vi "ThermoV_ControlSweep_2VO_160718.vi"() -> ()   [LabVIEW 2013]
uses:
  <vilib>/Analysis/baseanly.llb/Mean (DBL).vi
  <vilib>/Analysis/NI_AALBase.lvlib
panel:
  out "time/(60*13) indicator":dbl
  out "VGate Mod10 indicator":dbl
  in  "Operate HVpp\nOutput Timer":bool caption="Reset"
  out "modular 13":dbl
  in  "Number of seconds for \neach HVpp case state":dbl=30.0
  out "Elapsed Time (s)":dbl
  out "DC Value":dbl[](array[numeric]) format="%#.6f"
  in  "Saving Avg?":bool
  in  "Filename":path=path "trial_1.lvm"
  in  "STOP":bool
  in  "Save Waveform":bool
  out "Peak2Peak V":dbl[](array[numeric])
  out "Waveform Chart":dynamicdata(graph)
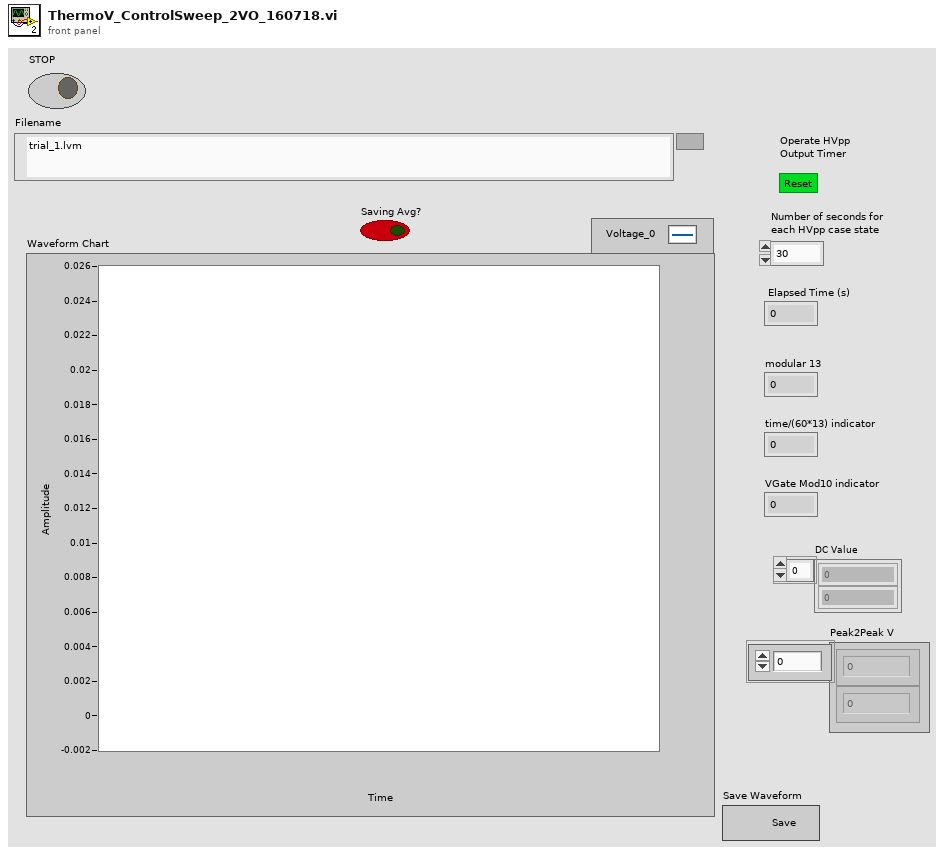
[diagram p1: front panel]
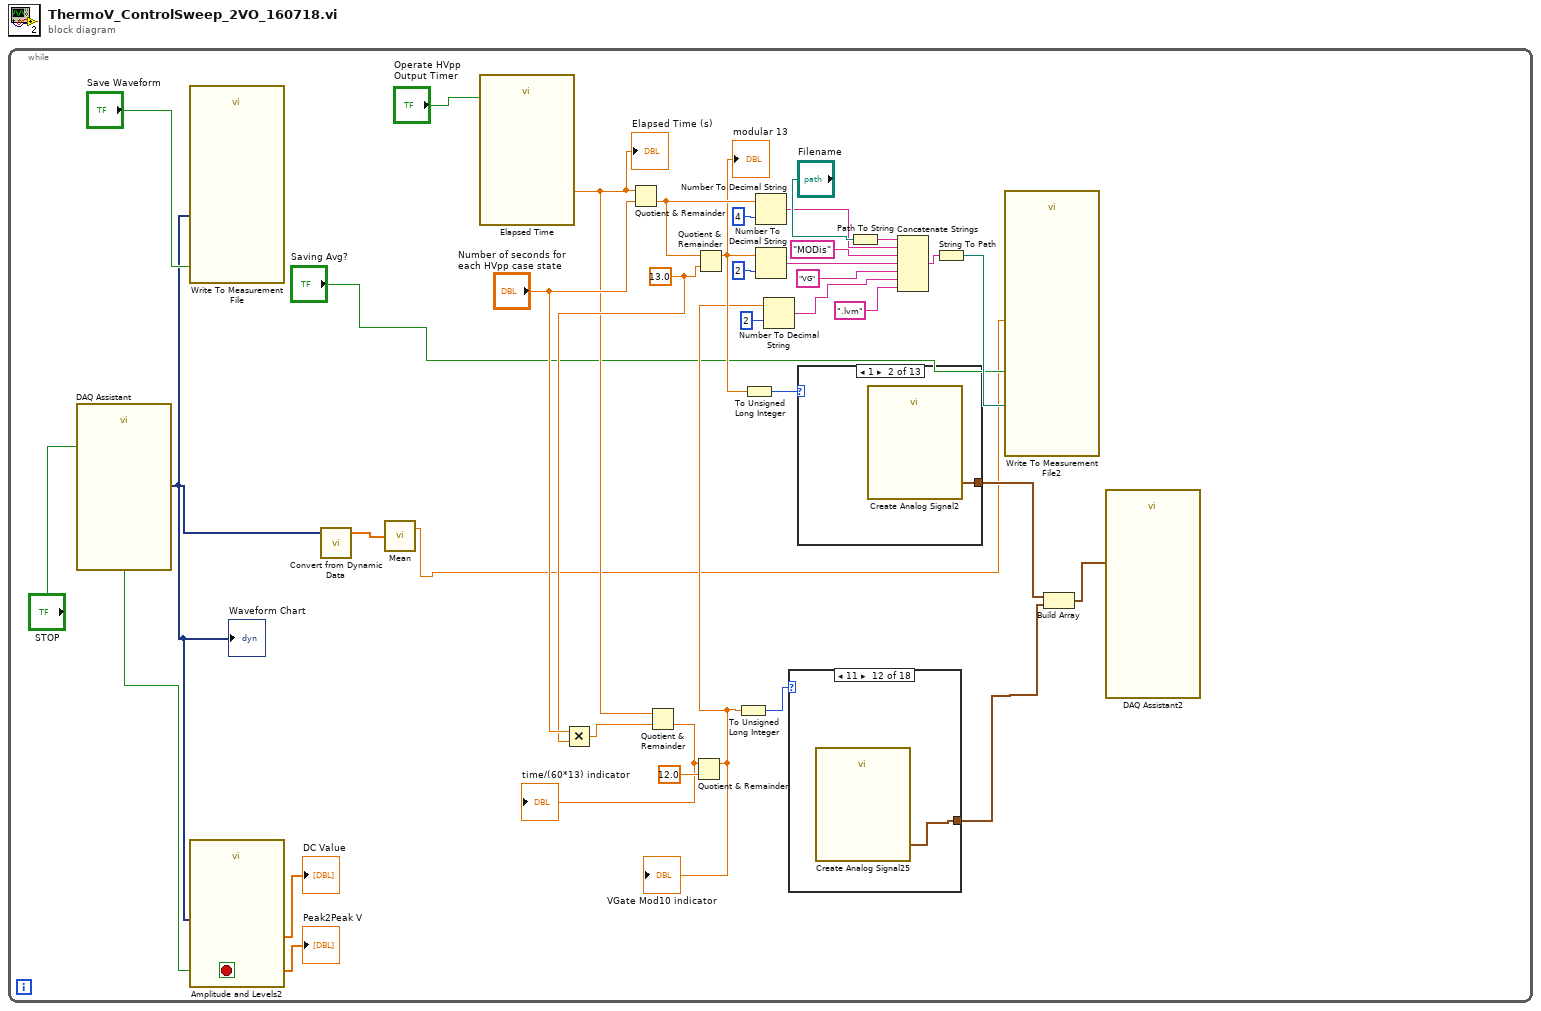
[diagram p0: block diagram]
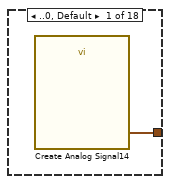
[diagram p2: hidden frame]
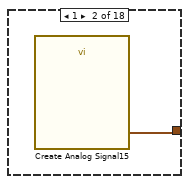
[diagram p3: hidden frame]
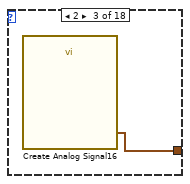
[diagram p4: hidden frame]
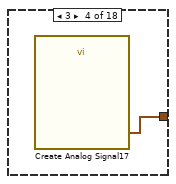
[diagram p5: hidden frame]
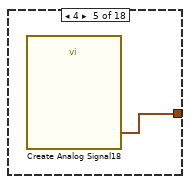
[diagram p6: hidden frame]
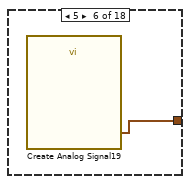
[diagram p7: hidden frame]
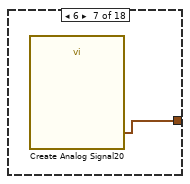
[diagram p8: hidden frame]
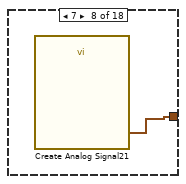
[diagram p9: hidden frame]
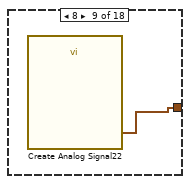
[diagram p10: hidden frame]
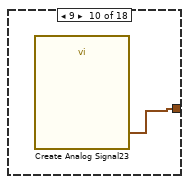
[diagram p11: hidden frame]
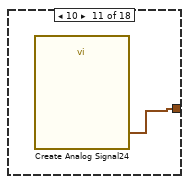
[diagram p12: hidden frame]
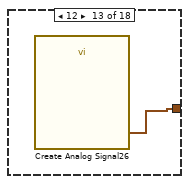
[diagram p13: hidden frame]
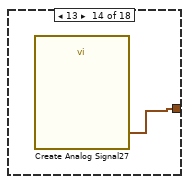
[diagram p14: hidden frame]
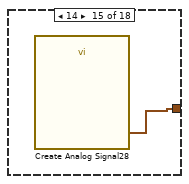
[diagram p15: hidden frame]
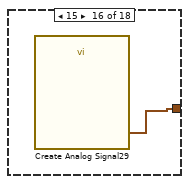
[diagram p16: hidden frame]
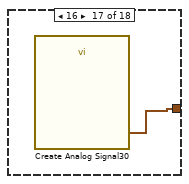
[diagram p17: hidden frame]
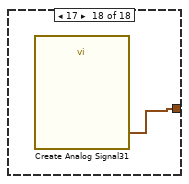
[diagram p18: hidden frame]
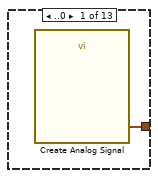
[diagram p19: hidden frame]
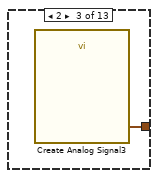
[diagram p20: hidden frame]
diagram:
  n1 = while {
    stop <- w37 stop-if-true
    w17 = 13.0 ("y")
    n2 = call "DAQ Assistant"("stop (F)"="STOP") -> ("data"=w3:dynamicdata, "stopped"=w37:bool)  [unwired: 15 in, 2 out]
    "Waveform Chart" <- w3
    n3 = call "Write To Measurement File"("Signals"=w3, "Enable"="Save Waveform") -> ()  [unwired: 15 in, 3 out]
    n4 = call "Amplitude and Levels2"("input signals"=w3) -> ("dc"=→"DC Value":dbl[], "peak-peak"=→"Peak2Peak V":dbl[])  [unwired: 15 in, 2 out]
    n5 = call "Convert from Dynamic Data"("Dynamic Data Type"=w3) -> ("Array"=w2:dbl[])  [unwired: 3 in]
    n6 = call-poly <vilib>:"Mean.vi"("X"=w2) -> ("mean"=w1:dbl)  [unwired: 1 out]
    n7 = call "Elapsed Time"("Reset"="Operate HVpp\nOutput Timer") -> ("Elapsed Time (s)"=w16:dbl)  [unwired: 11 in, 7 out]
    "Elapsed Time (s)" <- w16
    n8 = Multiply(x="Number of seconds for \neach HVpp case state", y=w17) -> (x*y=w19:dbl)
    n9 = Quotient & Remainder(x=w16, y="Number of seconds for \neach HVpp case state") -> (floor(x/y)=w26:dbl)  [unwired: 1 out]
    n10 = Quotient & Remainder(x=w16, y=w19) -> (floor(x/y)=w10:dbl)  [unwired: 1 out]
    "time/(60*13) indicator" <- w10
    n11 = Quotient & Remainder(x=w10, y=12.0) -> (x-y*floor(x/y)=w9:dbl)  [unwired: 1 out]
    "VGate Mod10 indicator" <- w9
    n12 = Quotient & Remainder(x=w26, y=w17) -> (x-y*floor(x/y)=w22:dbl)  [unwired: 1 out]
    "modular 13" <- w22
    n13 = To Unsigned Long Integer(number=w9) -> (unsigned 32bit integer=w15:u32)
    n14 = To Unsigned Long Integer(number=w22) -> (unsigned 32bit integer=w32:u32)
    n15 = Number To Decimal String(number=w26, width (-)=i16 4) -> (decimal integer string=w25:string)
    n16 = Number To Decimal String(number=w22, width (-)=i16 2) -> (decimal integer string=w21:string)
    n17 = Number To Decimal String(number=w9, width (-)=i16 2) -> (decimal integer string=w12:string)
    n18 = case shown="11" w15 {
      tunnel: [w38 w39 w40 w41 w42 w43 w44 w45 w46 w47 w48 w49 w50 w51 w52 w53 w54 w55] -> w7
      frame ..0, Default {
        n19 = call "Create Analog Signal14"() -> ("DC signal"=w38:waveform(dbl))  [unwired: 18 in, 1 out]
      }
      frame 1 {
        n20 = call "Create Analog Signal15"() -> ("DC signal"=w39:waveform(dbl))  [unwired: 18 in, 1 out]
      }
      frame 2 {
        n21 = call "Create Analog Signal16"() -> ("DC signal"=w40:waveform(dbl))  [unwired: 18 in, 1 out]
      }
      frame 3 {
        n22 = call "Create Analog Signal17"() -> ("DC signal"=w41:waveform(dbl))  [unwired: 18 in, 1 out]
      }
      frame 4 {
        n23 = call "Create Analog Signal18"() -> ("DC signal"=w42:waveform(dbl))  [unwired: 18 in, 1 out]
      }
      frame 5 {
        n24 = call "Create Analog Signal19"() -> ("DC signal"=w43:waveform(dbl))  [unwired: 18 in, 1 out]
      }
      frame 6 {
        n25 = call "Create Analog Signal20"() -> ("DC signal"=w44:waveform(dbl))  [unwired: 18 in, 1 out]
      }
      frame 7 {
        n26 = call "Create Analog Signal21"() -> ("DC signal"=w45:waveform(dbl))  [unwired: 18 in, 1 out]
      }
      frame 8 {
        n27 = call "Create Analog Signal22"() -> ("DC signal"=w46:waveform(dbl))  [unwired: 18 in, 1 out]
      }
      frame 9 {
        n28 = call "Create Analog Signal23"() -> ("DC signal"=w47:waveform(dbl))  [unwired: 18 in, 1 out]
      }
      frame 10 {
        n29 = call "Create Analog Signal24"() -> ("DC signal"=w48:waveform(dbl))  [unwired: 18 in, 1 out]
      }
      frame 11 {
        n30 = call "Create Analog Signal25"() -> ("DC signal"=w49:waveform(dbl))  [unwired: 18 in, 1 out]
      }
      frame 12 {
        n31 = call "Create Analog Signal26"() -> ("DC signal"=w50:waveform(dbl))  [unwired: 18 in, 1 out]
      }
      frame 13 {
        n32 = call "Create Analog Signal27"() -> ("DC signal"=w51:waveform(dbl))  [unwired: 18 in, 1 out]
      }
      frame 14 {
        n33 = call "Create Analog Signal28"() -> ("DC signal"=w52:waveform(dbl))  [unwired: 18 in, 1 out]
      }
      frame 15 {
        n34 = call "Create Analog Signal29"() -> ("DC signal"=w53:waveform(dbl))  [unwired: 18 in, 1 out]
      }
      frame 16 {
        n35 = call "Create Analog Signal30"() -> ("DC signal"=w54:waveform(dbl))  [unwired: 18 in, 1 out]
      }
      frame 17 {
        n36 = call "Create Analog Signal31"() -> ("DC signal"=w55:waveform(dbl))  [unwired: 18 in, 1 out]
      }
    }
    n37 = case shown="1" w32 {
      tunnel: [w56 w57 w58 w59 w60 w61 w62 w63 w64 w65 w66 w67 w68] -> w8
      frame ..0 {
        n38 = call "Create Analog Signal"() -> ("sine wave"=w56:waveform(dbl))  [unwired: 18 in, 1 out]
      }
      frame 1 {
        n39 = call "Create Analog Signal2"() -> ("sine wave"=w57:waveform(dbl))  [unwired: 18 in, 1 out]
      }
      frame 2 {
        n40 = call "Create Analog Signal3"() -> ("sine wave"=w58:waveform(dbl))  [unwired: 18 in, 1 out]
      }
      frame 3 {
        n41 = call "Create Analog Signal4"() -> ("sine wave"=w59:waveform(dbl))  [unwired: 18 in, 1 out]
      }
      frame 4 {
        n42 = call "Create Analog Signal5"() -> ("sine wave"=w60:waveform(dbl))  [unwired: 18 in, 1 out]
      }
      frame 5 {
        n43 = call "Create Analog Signal6"() -> ("sine wave"=w61:waveform(dbl))  [unwired: 18 in, 1 out]
      }
      frame 6 {
        n44 = call "Create Analog Signal7"() -> ("sine wave"=w62:waveform(dbl))  [unwired: 18 in, 1 out]
      }
      frame 7 {
        n45 = call "Create Analog Signal8"() -> ("sine wave"=w63:waveform(dbl))  [unwired: 18 in, 1 out]
      }
      frame 8 {
        n46 = call "Create Analog Signal9"() -> ("sine wave"=w64:waveform(dbl))  [unwired: 18 in, 1 out]
      }
      frame 9 {
        n47 = call "Create Analog Signal10"() -> ("sine wave"=w65:waveform(dbl))  [unwired: 18 in, 1 out]
      }
      frame 10 {
        n48 = call "Create Analog Signal11"() -> ("sine wave"=w66:waveform(dbl))  [unwired: 18 in, 1 out]
      }
      frame 11 {
        n49 = call "Create Analog Signal12"() -> ("sine wave"=w67:waveform(dbl))  [unwired: 18 in, 1 out]
      }
      frame 12.. {
        n50 = call "Create Analog Signal13"() -> ("sine wave"=w68:waveform(dbl))  [unwired: 18 in, 1 out]
      }
    }
    n51 = Path To String(path="Filename") -> (string=w28:string)
    n52 = Concatenate Strings(w28, w25, "MODis" ("string"), w21, "VG" ("string"), w12, ".lvm" ("string")) -> (w29:string)
    n53 = String To Path(string=w29) -> (path=w30:path)
    n54 = call "Write To Measurement File2"("Signals"=w1, "Enable"="Saving Avg?", "Filename"=w30) -> ()  [unwired: 14 in, 3 out]
    n55 = Build Array(w8, w7) -> (w6:waveform(dbl)[])
    n56 = call "DAQ Assistant2"("data"=w6) -> ()  [unwired: 16 in, 3 out]
  }
